vi "ChartsAndGraphs-unfinished.vi"() -> ()   [LabVIEW 2014]
uses:
  <vilib>/ptbypt/NI_PtbyPt.lvlib
panel:
  out "Waveform Graph":waveform(dbl)(graph)
  out "Waveform Chart":dbl(graph)
  in  "stop":bool
  in  "time step (s)":dbl=0.25
  in  "phase":dbl format="%0.2f"
  in  "frequency":dbl=0.5 format="%0.2f"
  in  "amplitude":dbl=1.0 format="%0.2f"
  # "Sine wave"
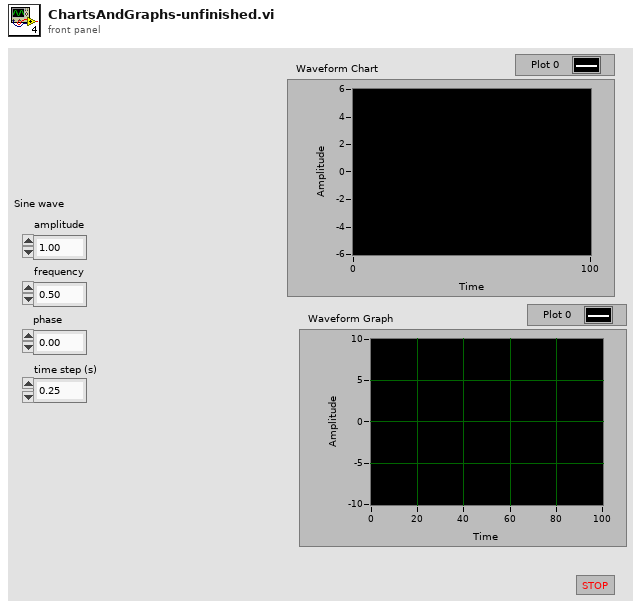
[diagram p1: front panel]
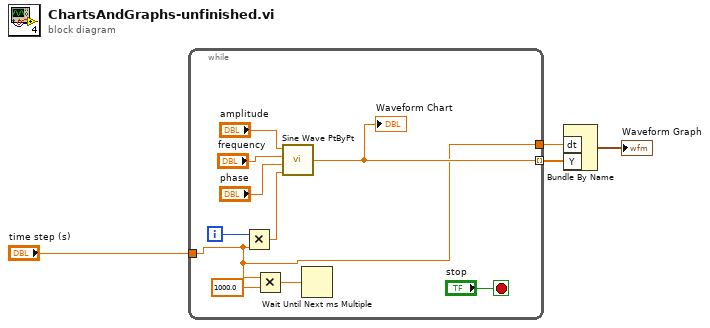
[diagram p0: block diagram]
diagram:
  n1 = while {
    tunnel: "time step (s)" -> [w5]
    tunnel: [w6] -> w3 mode=indexing
    tunnel: [w5] -> w2
    i -> [w10]
    stop <- "stop" stop-if-true
    n2 = Multiply(x=w10, y=w5) -> (x*y=w9:dbl)
    n3 = Multiply(x=w5, y=1000.0) -> (x*y=w7:dbl)
    n4 = call <vilib>:"Sine Wave PtByPt.vi"("time"=w9, "phase"="phase", "frequency"="frequency", "amplitude"="amplitude") -> ("sine wave"=w6:dbl)
    "Waveform Chart" <- w6
    n5 = Wait Until Next ms Multiple(millisecond multiple=w7) -> ()  [unwired: 1 out]
  }
  n6 = Bundle By Name("dt"=w2, "Y"=w3) -> (→"Waveform Graph":waveform(dbl))  [unwired: 1 in]
